vi "CreateModuleBroadcasts.vi"(8 "error in (no error)":errorcluster) -> (0 "error out":errorcluster, 3 "Broadcasts":T1)   [LabVIEW 2024, in "TesterModule.lvclass"]
uses:
  TesterModule.lvclass
  Broadcast Events--cluster.ctl
  Stopped.ctl
  TesterModule.lvclass/TesterModule.ctl
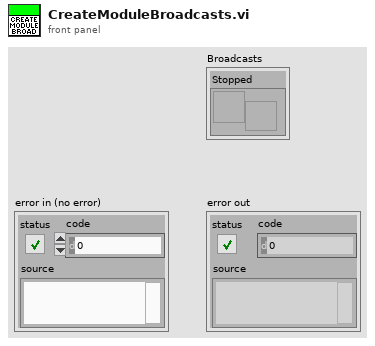
[diagram p1: front panel]
types:
  T1 = typedef "TesterModule.lvclass/Broadcast Events--cluster.ctl" = cluster{"Stopped":refnum<user-event>}
  T2 = typedef "TesterModule.lvclass/Stopped.ctl" = bool
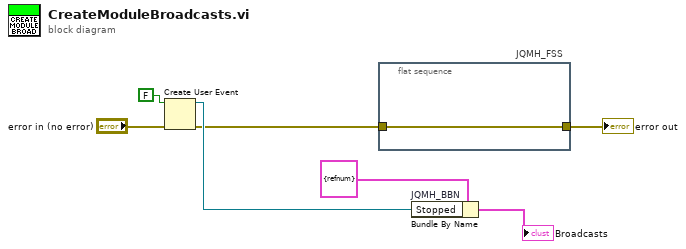
[diagram p0: block diagram]
diagram:
  n1 = Create User Event(user event datatype=T2 FALSE ("Stopped"), error in="error in (no error)") -> (user event=w6:refnum<user-event>, error out=w1:errorcluster)
  n2 = flat-sequence "JQMH_FSS" {
    tunnel: w1 -> [w8]
    tunnel: [w8] -> w2
    frame #0 {
    }
  }
  n3 = Bundle By Name "JQMH_BBN"(cluster=T1 {"Stopped"=refnum} ("Broadcasts"), "Stopped"=w6) -> (→"Broadcasts":T1)
  "error out" <- w2
